vi "Write Voltaje.vi"(8 "error in (no error)":errorcluster, 10 "Voltaje":dbl, 11 "Fuente de poder in":refnum<class "Fuente de poder.lvclass">) -> (0 "error out":errorcluster, 3 "Fuente de poder out":refnum<class "Fuente de poder.lvclass">)   [LabVIEW 2020, in "Fuente de poder.lvclass"]
uses:
  Fuente de poder.lvclass
  Fuente de poder.lvclass/Fuente de poder.ctl
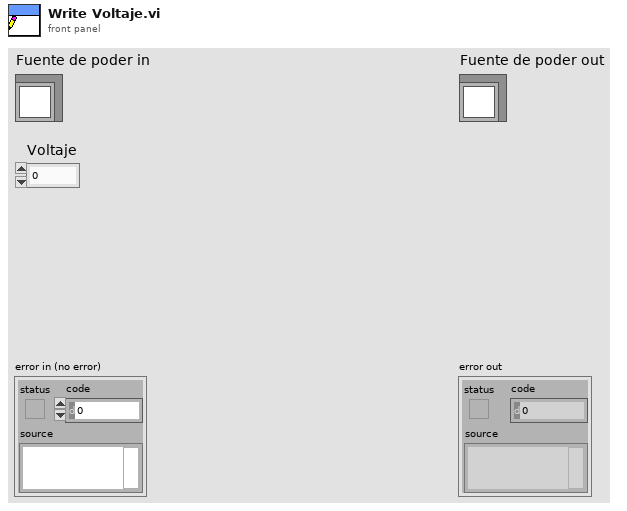
[diagram p1: front panel]
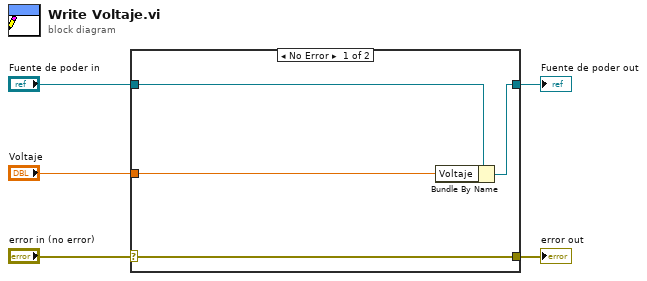
[diagram p0: block diagram]
diagram:
  n1 = case shown="No Error" "error in (no error)" {
    selector: "error in (no error)" -> [w9 w10]
    tunnel: [w9 w10] -> w4
    tunnel: [w7 w11] -> w2
    tunnel: "Fuente de poder in" -> [w8 w11]
    tunnel: "Voltaje" -> [w6 _]
    frame No Error {
      n2 = Bundle By Name(cluster=w8, "Voltaje"=w6) -> (w7:refnum<class "Fuente de poder.lvclass">)
    }
    frame Error {
    }
  }
  "error out" <- w4
  "Fuente de poder out" <- w2
